vi "Parse.vi"(8 "Error In":errorcluster, 11 "object in":refnum<class "2024_1.lvclass">) -> (0 "Error Out":errorcluster, 3 "object out":refnum<class "2024_1.lvclass">)   [LabVIEW 2023, in "2024_1.lvclass"]
uses:
  2024_1.lvclass
  2024_1.lvclass/2024_1.ctl
  <vilib>/Utility/error.llb/Trim Whitespace One-Sided.vi
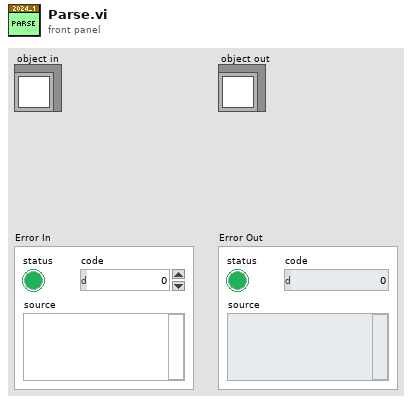
[diagram p1: front panel]
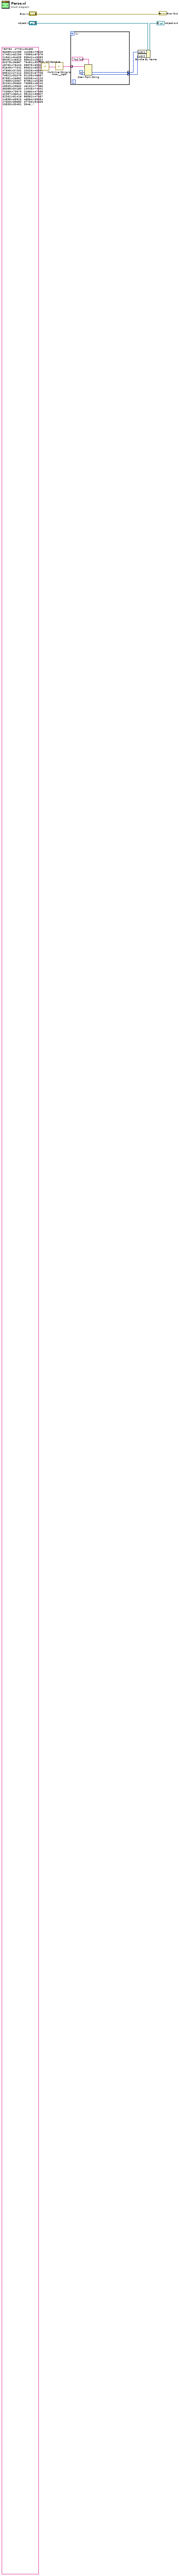
[diagram p0: block diagram]
diagram:
  n1 = call <vilib>:"Trim Whitespace.vi"("string"="80784   47731\n81682   36089\n22289   41038\n79525   17481\n62156   70590\n87975   21561\n54635   59542\n43393   99451\n45310   59542\n18324   92078\n36887   79481\n35723   48782\n78420   35875\n93307   52649\n77342   80601\n69125   47895\n37292   20025\n45553   59542\n27412   30010\n67708   70822\n92078   91109\n48367   87581\n26852   30538\n42123   17859\n20067   87581\n20239   32262\n50660   73585\n46240   45533\n29502   46131\n77080   36089\n64180   14043\n74942   72085\n73979   22860\n47999   41397\n36014   35101\n39827   32262\n81418   86581\n47467   14538\n65923   46584\n95054   17500\n59680   37730\n94609   19539\n33451   39467\n69173   12422\n31769   34255\n85180   29056\n82104   52296\n90955   38171\n83927   70590\n59455   17306\n28681   86581\n54107   13789\n79824   21386\n53890   46519\n94883   87581\n12797   46584\n66809   24306\n78327   24086\n19780   43234\n55623   38171\n10937   42288\n24262   74556\n92076   77080\n69179   15029\n13764   52214\n92187   63803\n91328   94609\n24356   36089\n82974   84225\n55924   70822\n65439   55383\n78097   82069\n58045   12422\n72087   37730\n70822   32262\n78511   48368\n39251   54157\n74623   59542\n32104   74623\n69499   17481\n97919   33260\n37778   74623\n56977   14684\n19100   98708\n29453   34463\n18839   87581\n75434   75839\n58303   84225\n84924   24108\n99813   37730\n99218   93749\n54262   38470\n61773   94274\n67034   56935\n71788   74556\n83455   22604\n76089   84225\n11003   85999\n80814   62471\n41928   56000\n52541   71034\n37488   53519\n78475   33260\n57117   32449\n54543   54732\n19050   52775\n80967   76950\n71045   29497\n61189   43136\n75055   38171\n91573   46131\n50100   70590\n46554   24973\n25154   99579\n19853   77080\n11807   20266\n40158   24315\n92543   38171\n93300   87581\n79628   68978\n19164   51702\n53719   96515\n38074   46503\n25693   53188\n79321   17481\n25108   21108\n38398   72487\n22073   59542\n98191   39605\n80619   66029\n99138   74556\n49897   33260\n84225   10112\n14331   66948\n94603   36089\n33642   75862\n14314   89669\n12998   48362\n10989   21312\n68074   46131\n10531   47636\n32312   70590\n66844   38171\n73563   77034\n33099   65439\n93734   71747\n56538   35101\n55501   82069\n19974   94609\n21308   23592\n37062   36089\n99908   59542\n92651   94321\n81371   84225\n96268   35101\n58685   25444\n37191   86819\n71956   87899\n28341   70822\n11995   64983\n92426   70590\n30515   57117\n72193   37685\n82150   77080\n19292   73860\n52076   53020\n26135   78522\n49482   79269\n56103   81747\n62006   66781\n41905   24906\n23782   10112\n39865   41627\n80074   91781\n84213   70822\n19586   43155\n87133   70822\n67811   65439\n60019   23478\n29057   70590\n77349   16491\n32372   13789\n93055   65439\n82209   30330\n75731   60775\n91276   79848\n90330   37730\n41180   59542\n81204   95937\n36092   11620\n13033   38171\n34488   51306\n71770   81668\n37630   57117\n87608   69809\n90593   59542\n52792   39467\n33508   46226\n78150   29434\n18072   84225\n11205   63803\n28801   39467\n89617   47552\n91269   77080\n50829   15405\n96387   68582\n44407   46131\n17491   74556\n77464   57117\n67053   71830\n67048   20722\n15369   76996\n71812   74803\n96980   35466\n39993   82069\n65498   59148\n88138   79430\n16497   54357\n75624   46131\n84028   39464\n82572   39122\n14297   36089\n33805   85723\n44778   74556\n14498   87581\n71384   17116\n47173   82069\n60652   82069\n67241   46316\n73276   80192\n46786   68313\n88795   97650\n95120   23939\n53010   82069\n40256   82069\n26913   71782\n44746   88309\n49866   86581\n50951   97892\n80832   30492\n22643   70822\n84334   86581\n96028   70590\n39816   56848\n78427   63379\n27147   92078\n35658   12422\n76747   47552\n32896   59542\n98898   12422\n45166   37081\n38602   27009\n17507   82069\n75567   74623\n71921   29970\n11800   90710\n23973   68582\n80315   68252\n86659   13782\n23014   71633\n33041   57117\n93351   65439\n69088   46584\n71994   91050\n61532   98835\n98790   76392\n62890   75035\n37723   36089\n56136   20455\n91663   84225\n76413   87581\n89223   11659\n33477   47973\n34541   16506\n82603   59542\n37730   75791\n25272   98835\n86703   82248\n56755   54948\n74556   92078\n11337   36089\n52534   27174\n60327   87581\n84554   89264\n11381   59542\n99601   81999\n20139   33278\n25530   59558\n97414   74906\n11269   70822\n66500   13789\n23195   68582\n22872   53300\n94937   51202\n12273   55687\n63364   71074\n14160   15554\n57473   39467\n19091   87899\n43286   16810\n25975   33571\n57319   39467\n61075   66766\n95980   98826\n47190   55086\n82297   87581\n24071   53175\n85766   82069\n48467   36089\n16301   77080\n89176   48368\n76512   29182\n61987   37730\n10252   83226\n42503   12203\n75498   71010\n56685   98679\n22338   48368\n40666   86581\n88276   32262\n69493   94854\n75435   22046\n91561   48368\n99202   42878\n90978   38171\n89712   77080\n48877   36148\n31528   92078\n15135   36258\n47468   10112\n23557   10112\n46381   98492\n95007   57390\n31053   95937\n26099   27278\n34939   75494\n44252   59542\n54945   73875\n26328   38171\n73116   46131\n16168   13789\n28518   28323\n25310   28056\n63436   27589\n77562   37730\n80614   82409\n76421   63235\n24521   53590\n17937   86492\n80687   56569\n56076   10767\n64810   74623\n73278   26540\n58083   46584\n90208   32262\n17793   65461\n92155   47552\n47982   91242\n82069   77080\n39226   87581\n34622   42348\n99735   46584\n22264   37730\n46131   70590\n90426   18162\n75148   63803\n98835   70822\n80373   30652\n62705   46131\n95974   32262\n54882   36453\n50578   71111\n30132   39798\n22527   35101\n41027   91852\n69013   46238\n79152   69190\n89330   61021\n85358   13789\n15086   54357\n50002   39467\n42579   42483\n11717   87581\n43825   24664\n50771   87581\n89105   45839\n84561   92078\n42692   38899\n20001   94609\n40205   38051\n13295   20519\n96020   10112\n47293   87899\n94929   10112\n24422   82448\n62066   59975\n52303   86581\n79329   72343\n69417   16516\n13062   47552\n41201   84658\n92635   62180\n19834   91848\n34343   18222\n18208   30134\n82611   63803\n12207   74511\n93804   53502\n51066   33260\n28374   66275\n34107   10112\n13223   80233\n97959   94470\n51054   57117\n82951   30540\n61626   32898\n52816   16045\n67095   46131\n96825   70590\n34307   77500\n98853   35083\n76437   65439\n71489   77080\n46520   16597\n15288   54357\n34660   63199\n65053   65439\n99414   57117\n85660   83055\n10245   32262\n12775   67705\n57298   65439\n64105   36878\n36104   12422\n89241   56000\n41045   87764\n16506   88026\n53044   44649\n17425   84939\n56000   69714\n63575   92078\n50418   19328\n39915   10112\n97542   66182\n97468   16506\n74779   94609\n90120   17677\n91404   87581\n83440   31253\n80583   16585\n16542   82069\n34305   48368\n95455   30383\n56639   87581\n33983   12422\n36565   47552\n63737   32262\n60378   37730\n80067   95189\n45068   61725\n20720   74180\n24918   94609\n18264   86581\n43293   57117\n67279   38551\n75286   95937\n19582   71378\n62806   12497\n48345   96497\n45026   68499\n97371   36028\n80754   74761\n97543   54357\n51110   12422\n23427   24635\n44698   68582\n84624   28102\n74813   12960\n94691   82069\n68498   93943\n30492   52810\n65243   34777\n12244   82069\n14525   65439\n75430   98694\n73494   87567\n97587   67336\n59739   59542\n38047   30492\n35519   43518\n64167   92078\n52460   72101\n49707   81573\n86581   24885\n93340   69244\n91249   13789\n35632   52637\n78007   56318\n86640   46131\n84853   30492\n69589   55403\n87840   94609\n15931   65439\n87788   94609\n36704   39467\n56849   92199\n23845   70822\n58771   59306\n15094   72864\n78669   38116\n67290   30492\n30809   12422\n60616   82069\n99946   86597\n57245   10112\n14346   59022\n95083   79436\n57974   65334\n22448   86581\n89557   42455\n72735   70224\n80323   28694\n19558   59542\n66100   67968\n29557   54357\n75549   48368\n47979   65120\n81370   26550\n99542   80446\n92151   48368\n60693   60658\n70590   36856\n93811   95439\n50263   78334\n51728   74556\n48629   23585\n63500   35242\n98688   74623\n50638   39467\n39320   57117\n85601   48368\n86749   63803\n84452   24596\n40346   33260\n56693   59543\n96450   10429\n46319   50421\n88183   63450\n47057   56000\n99066   65734\n95736   95937\n49970   77187\n76310   86581\n72960   21713\n61234   33798\n20364   70590\n89304   82069\n90141   11734\n11708   88748\n67064   10112\n51923   71970\n47055   36089\n45990   28498\n89727   87581\n92801   71911\n39807   46584\n72390   35136\n16446   62868\n77863   56000\n42686   13789\n28678   75289\n84858   67442\n64404   84225\n77138   70822\n48368   33260\n89589   10112\n92469   43286\n66906   19599\n96794   74623\n98997   15262\n32791   74556\n86217   36089\n23368   31640\n88661   19276\n72933   85540\n22703   30492\n71905   65439\n58050   40461\n29588   95734\n39243   55933\n83527   17481\n15249   58026\n77033   47662\n47552   86581\n57262   69752\n20061   18772\n81279   43751\n58632   70157\n13683   94609\n21964   74556\n95224   59604\n83465   88283\n81225   36089\n16585   17481\n15766   15653\n50261   57292\n82233   54937\n60140   94609\n52750   31767\n20808   56000\n57243   92469\n43252   32262\n60198   86581\n18620   55678\n44051   50219\n15210   39162\n60005   36089\n66217   74556\n13853   70822\n63803   70822\n35040   65079\n65842   38038\n39316   20720\n87663   65984\n20060   68582\n25890   48796\n16116   82639\n31571   70822\n43980   84152\n53704   11951\n79055   42179\n57231   22127\n88376   85408\n59541   95959\n92556   53432\n88194   16317\n34727   30904\n16387   57117\n96730   10644\n65083   36089\n15228   16506\n81423   59542\n87899   17481\n90911   85798\n17159   83599\n50392   77080\n22864   43286\n37528   94609\n21429   59542\n28265   46877\n46764   37608\n91323   65439\n83391   35269\n74503   39369\n93683   63803\n31047   38528\n53705   33260\n74884   86581\n54241   99733\n45641   73338\n64783   94609\n36885   76835\n94878   70590\n95560   21274\n61985   67119\n65075   74623\n32813   86204\n36749   72304\n78654   50542\n86690   74556\n70019   32262\n20641   60329\n77752   57117\n60383   20123\n90352   74623\n24141   71761\n65390   10350\n47054   38708\n39003   57915\n38161   92078\n38171   32262\n84400   10112\n15341   70822\n39428   16506\n13942   13789\n96936   70483\n93060   50175\n38192   67104\n46944   64882\n10846   12422\n35101   35801\n91104   20720\n13040   13789\n32161   31456\n97253   86581\n70362   70590\n53579   26550\n32295   56680\n77624   74556\n19453   38171\n11458   82069\n39312   94596\n68109   81118\n63009   59542\n96761   33260\n42532   96201\n42166   87800\n87613   44967\n69532   34024\n48387   83207\n54987   28919\n20342   84225\n23664   56000\n46174   10112\n72309   12474\n72157   73250\n28932   14632\n36882   84225\n23261   38171\n99849   41962\n95036   44159\n67696   12422\n58158   12422\n99688   84696\n95937   56267\n67472   28880\n32262   78595\n39793   31505\n53311   87581\n28411   51506\n53156   88986\n97772   95152\n27795   70590\n25013   30223\n14528   72611\n76358   11601\n46584   32226\n45091   53888\n78740   82069\n28185   56000\n86150   33260\n12422   13789\n49946   36089\n39558   91418\n12969   78072\n30758   23674\n30625   72335\n29062   46065\n51088   61952\n88725   61869\n94002   74556\n35800   29768\n43599   95937\n65922   82638\n52159   91936\n96552   48368\n29575   38995\n51418   82069\n39467   36420\n76259   15058\n52506   24873\n34793   68305\n36089   94116\n25337   69496\n46924   86581\n62992   82069\n62236   95937\n50926   25384\n72595   74556\n53666   67031\n44374   15724\n44629   51188\n80493   95937\n76680   59202\n96833   95937\n96740   86581\n90400   65439\n41922   10112\n10333   23762\n13789   94609\n79941   85091\n34855   55865\n87532   37140\n85678   46584\n34735   74556\n27059   28517\n62170   92078\n59542   84972\n44107   46131\n62531   86581\n36662   56000\n36292   59542\n76115   57037\n39296   41740\n34919   10743\n74948   86439\n50539   59294\n85056   31471\n28116   65439\n39085   38176\n84409   95937\n57138   46131\n72483   57117\n32395   72441\n95005   74883\n87581   51660\n28602   28664\n34996   46131\n96430   56339\n77226   70822\n93760   10112\n40364   94609\n40141   39467\n68490   40042\n48192   93216\n68068   70590\n73633   15355\n83619   47552\n81572   73873\n25924   70822\n29554   63803\n19515   26687\n61203   65439\n66108   77080\n34039   33260\n54877   35542\n38583   96489\n90667   42450\n84938   10487\n46965   59542\n54823   74069\n71321   73685\n19154   57117\n73217   30492\n76105   13647\n39670   12422\n30004   64951\n21400   16931\n58732   46131\n46185   57117\n35140   97447\n21937   32262\n29766   37730\n97110   17481\n37622   70822\n10481   46131\n89082   37730\n37941   74556\n14004   13789\n75256   31754\n91586   98835\n70127   84728\n27519   76800\n30742   29667\n40956   72181\n38337   85286\n93338   32262\n17167   48368\n90586   87581\n77695   72650\n78449   10112\n14007   92469\n44816   56000\n92128   12422\n70434   89508\n46495   17481\n86412   57117\n12915   29947\n31239   98835\n25873   62842\n18560   54357\n56101   27741\n85775   70590\n36475   51980\n80038   10112\n98826   30492\n41315   82816\n11389   82624\n11947   75881\n26407   10112\n30869   41026\n87026   44676\n41060   77177\n27239   32212\n50309   47552\n28120   35101\n52772   87899\n50851   13789\n52738   67642\n73374   61276\n29063   83110\n75283   77080\n91345   33260\n14809   19229\n82519   27777\n92688   65439\n10526   48368\n59702   92469\n35688   48965\n87590   24828\n40206   75331\n36194   74556\n43336   12746\n26034   29117\n23466   47552\n33234   19772\n17481   11383\n68582   54357\n36038   20809\n33704   98835\n87642   46131\n37947   38171\n17577   54357\n13994   48368\n70913   45734\n11985   23504\n82269   84225\n83126   70590\n47981   50609\n71785   10112\n38305   87857\n59774   78056\n62970   82069\n21547   84225\n63443   87640\n74676   92894\n54357   35752\n88456   38171\n80643   40334\n78727   73557\n86551   13789\n31360   70822\n38144   12422\n39925   26550\n18733   67964\n14557   23598\n68231   70590\n28923   37251\n36731   36089\n16989   57160\n10112   90976\n81269   32323\n46176   11467\n34165   74556\n30496   32262\n33260   70590\n91319   45070\n80484   38171\n61567   48368\n36103   70590\n45693   70590\n41025   43757\n36802   65596\n21523   98958\n80599   32262\n49397   92078\n74366   65439\n30292   94948\n20673   10112\n13158   46131\n89970   26550\n70825   12276\n96736   32750\n26698   17481\n94201   26049\n66228   18185\n50623   91018\n63509   70822\n96572   46131\n34380   46715\n21120   17481\n24159   56000\n59659   74556\n31572   53951\n48375   82069\n12985   36089\n82040   10557\n63252   57117\n31520   86581\n38262   13789\n41980   40901\n76273   47552\n11812   46131\n28759   77080\n12882   92653\n64935   33260\n26550   83813\n19156   58394\n93914   35101\n43129   96976\n13090   57117\n98463   76524\n36993   46131\n89249   35207\n12936   18458\n26497   56000\n75288   35237\n79742   82354\n65715   12422\n21544   29737" ("PuzzleInput")) -> ("trimmed string"=w4:string)  [unwired: 1 in]
  n2 = call <userlib>:"Multi-line String to Array__ogtk.vi"("string"=w4) -> ("lines"=w3:string[])
  n3 = for {
    tunnel: w3 -> [w13] mode=indexing
    tunnel: [w11] -> w2 mode=indexing
    tunnel: [w10] -> w1 mode=indexing
    w9 = i64 0 ("default value 1")
    n4 = Scan From String(format string="%d %d", input string=w13, default 1=w9, default 2=w9) -> (output 1=w11:i64, output 2=w10:i64)  [unwired: 2 in, 3 out]
  }
  n5 = Bundle By Name(cluster="object in", "List 1"=w2, "List 2"=w1) -> (→"object out":refnum<class "2024_1.lvclass">)
  "Error Out" <- "Error In"
